vi "Close_LTA-HS.vi"(11 "Connection Cluster in":T1) -> (0 "error out":errorcluster)   [LabVIEW 2013]
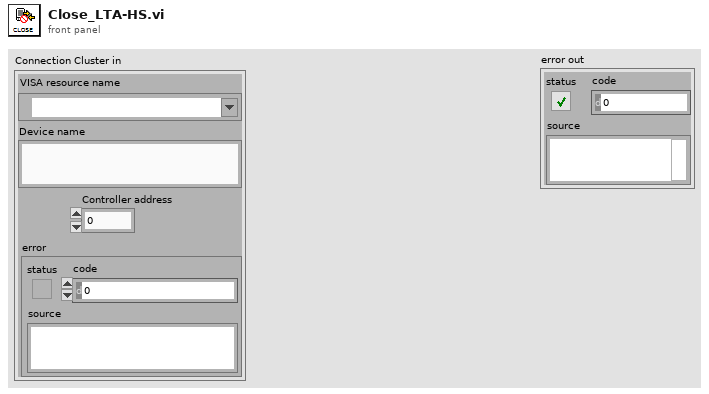
[diagram p1: front panel]
types:
  T1 = cluster{"VISA resource name":refnum<visa-resource-name>, "Device name":string, "Controller address":i32, "error":errorcluster}
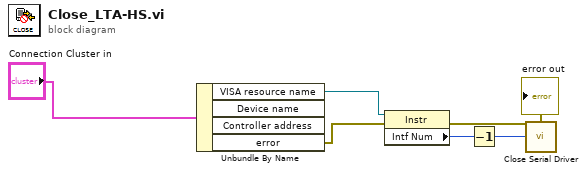
[diagram p0: block diagram]
diagram:
  n1 = Unbundle By Name("Connection Cluster in") -> ("VISA resource name"=w3:refnum<visa-resource-name>, "error"=w2:errorcluster)  [unwired: 2 out]
  n2 = property class="Instr"(reference=w3, error in=w2) -> (error out=→"error out":errorcluster, "Intf Num"=w6:u16)  [unwired: 1 out]
  n3 = Decrement(x=w6) -> (x-1=w5:u16)
  n4 = call <vilib>:"Close Serial Driver.vi"("port number"=w5) -> ()  [unwired: 1 out]
